vi "Connect.vi"(8 "error in (no error)":errorcluster, 9 "ConfigDir":u8[](array[numeric])=array[4097 elements], 10 "nSensorIP":u32, 11 "nHostIP":u32) -> (0 "error out":errorcluster, 3 "function return":i32)   [LabVIEW 2022 SP3, in "BonTechDetector.lvlib"]
doc: "extern \"C\" BONTECHLIBRARY_API int __stdcall Connect(unsigned int nHostIP, unsigned int nSensorIP, LPTSTR ConfigDir);"
uses:
  BonTechDetector.lvlib
  BonTechWrapperLibrary.dll
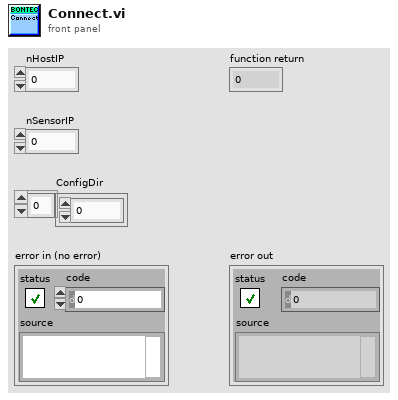
[diagram p1: front panel]
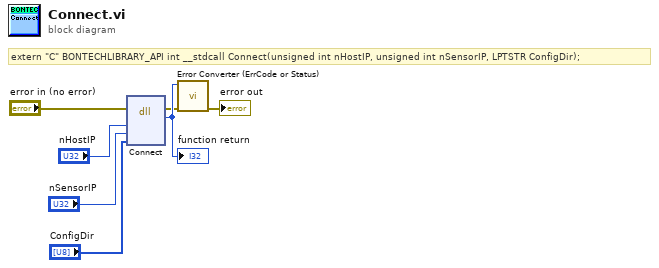
[diagram p0: block diagram]
diagram:
  # "extern \"C\" BONTECHLIBRARY_API int __stdcall Connect(unsigned int nHostIP, unsigned int nSensorIP, LPTSTR ConfigDir);"
  n1 = dll-call lib="E:/Workspace/The-Oracle-feature-highlight-smooth-filter-on-freeze-mode/Image Acquisition/Child Classes/BonTechFlatPanel/BonTechWrapperLibrary.*" fn="Connect"(error in="error in (no error)", "nHostIP"="nHostIP", "nSensorIP"="nSensorIP", "ConfigDir"="ConfigDir") -> (error out=w2:errorcluster, "return type"=w7:i32)  [unwired: 5 in, 1 out]
  "function return" <- w7
  n2 = call "Error Converter (ErrCode or Status).vi"("error in (no error)"=w2, "error code"=w7) -> ("error out"=→"error out":errorcluster)  [unwired: 9 in]
